vi "Read timeout.vi"(11 "Properties.Suite in":refnum<class "Properties.Suite.lvclass">) -> (2 "timeout":i32=1000, 3 "Properties.Suite out":refnum<class "Properties.Suite.lvclass">)   [LabVIEW 2013, in "Caraya.lvlib" / "Properties.Suite.lvclass"]
uses:
  Properties.Suite.lvclass
  Properties.Suite.lvclass/Properties.Suite.ctl
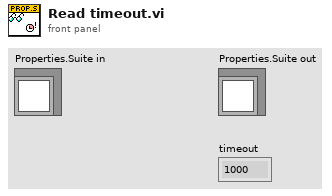
[diagram p1: front panel]
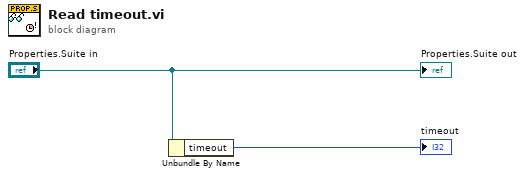
[diagram p0: block diagram]
diagram:
  n1 = Unbundle By Name("Properties.Suite in") -> ("timeout"=→"timeout":i32)
  "Properties.Suite out" <- "Properties.Suite in"
